vi "GetDir.vi"() -> (0 "Project Directory (../)":path, 1 "Documentation Directory (../doc/)":path, 2 "Image Directory (../doc/img/)":path)   [LabVIEW 2017, in "DocTools.lvlib"]
uses:
  DocTools.lvlib
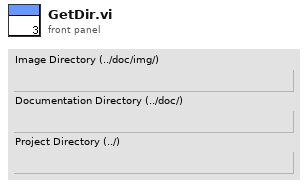
[diagram p1: front panel]
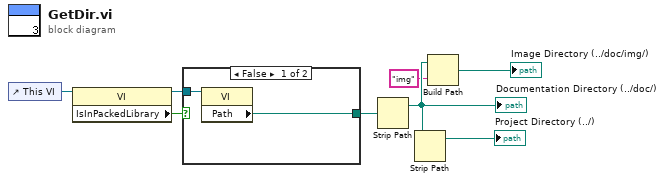
[diagram p0: block diagram]
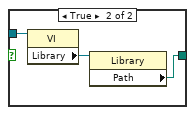
[diagram p2: hidden frame]
diagram:
  n1 = control-ref of="This VI"() -> (w8:refnum<vi>)
  n2 = property class="VI"(reference=w8) -> (reference out=w6:refnum<vi>, "IsInPackedLibrary"=w7:bool)  [unwired: 1 in, 1 out]
  n3 = case shown="False" w7 {
    tunnel: w6 -> [w10 w13]
    tunnel: [w9 w11] -> w5
    frame False {
      n4 = property class="VI"(reference=w10) -> ("Path"=w9:path)  [unwired: 1 in, 2 out]
    }
    frame True {
      n5 = property class="VI"(reference=w13) -> ("Library"=w12:refnum<vi>)  [unwired: 1 in, 2 out]
      n6 = property class="Library"(reference=w12) -> ("Path"=w11:path)  [unwired: 1 in, 2 out]
    }
  }
  n7 = Strip Path(path=w5) -> (stripped path=w3:path)  [unwired: 1 out]
  "Documentation Directory (../doc/)" <- w3
  n8 = Strip Path(path=w3) -> (stripped path=→"Project Directory (../)":path)  [unwired: 1 out]
  n9 = Build Path(base path=w3, name or relative path="img") -> (appended path=→"Image Directory (../doc/img/)":path)
